vi "Get Anonynous Credentials.vi"() -> (0 "Anonymous password":string, 2 "Anonymous username":string)   [LabVIEW 2013, in "Connection_GOSPL.lvlib" / "Store.lvclass"]
uses:
  Store.lvclass
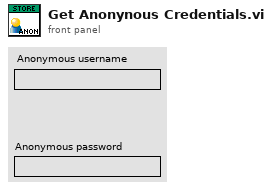
[diagram p1: front panel]
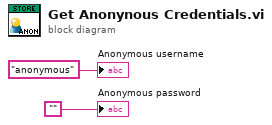
[diagram p0: block diagram]
diagram:
  "Anonymous username" <- "anonymous" ("Anonymous username")
  "Anonymous password" <- ""
